vi "Read files V(Delay).vi"(10 "Path":path, 11 "Number":dbl) -> (3 "V":dbl format="%#_1g")   [LabVIEW 2020, in "GPP.lvlib"]
uses:
  GPP.lvlib
panel:
  out "V1":string
  out "Time":string
  out "LAST1":string
  out "Voltege":string
  out "ALL":string
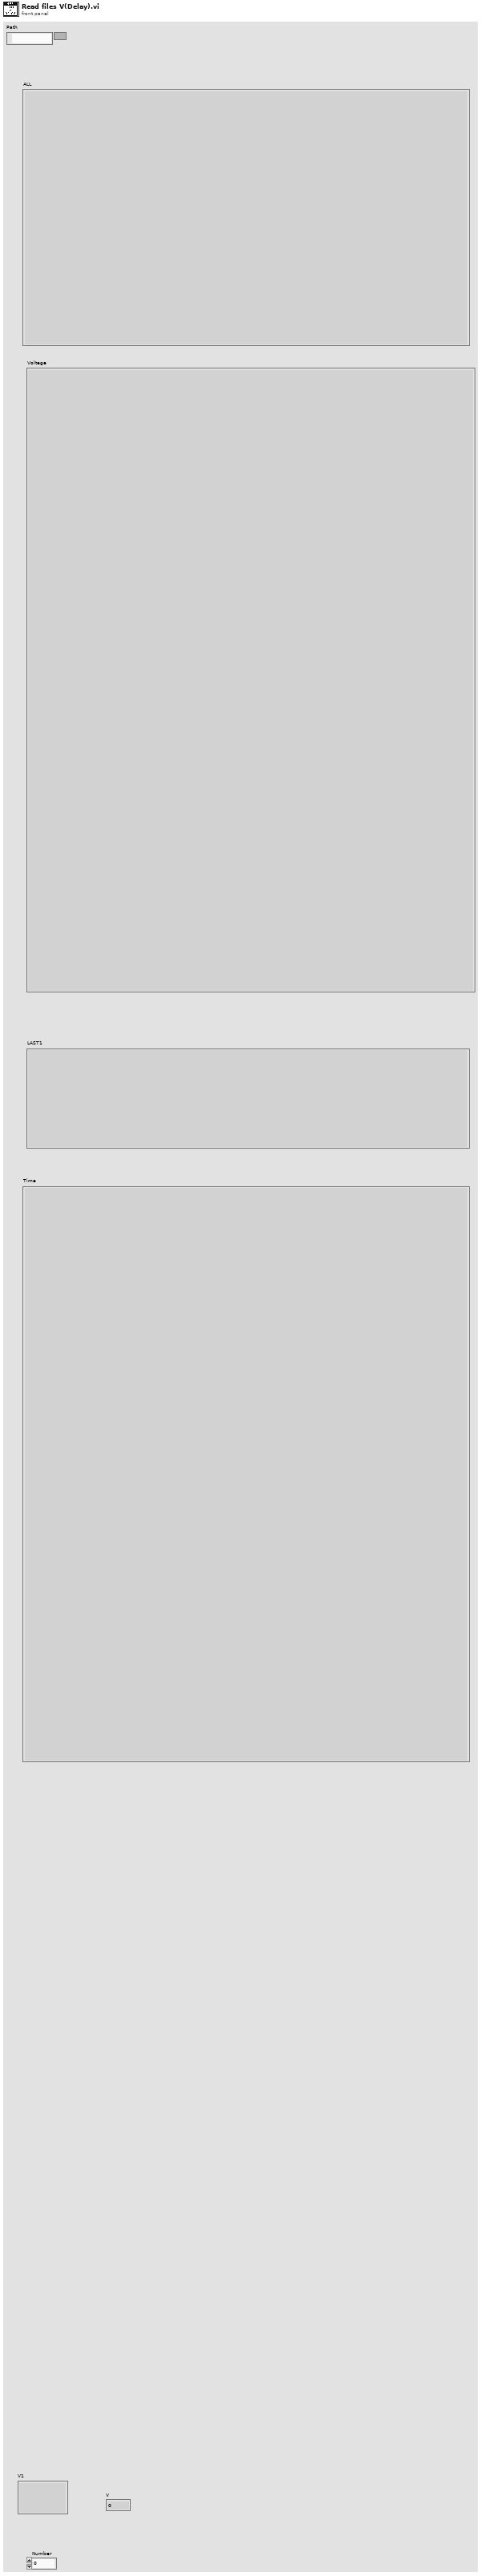
[diagram p1: front panel]
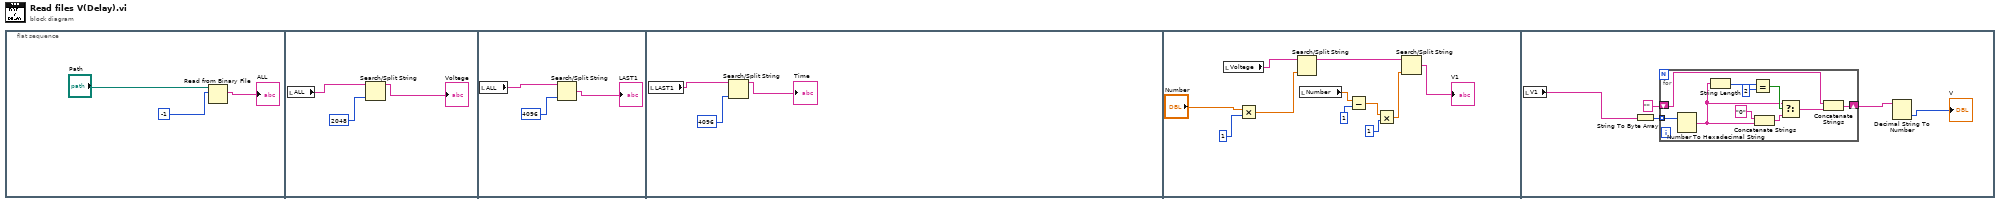
[diagram p0: block diagram]
diagram:
  n1 = flat-sequence {
    frame #0 {
      n2 = Read from Binary File(10:-1, 11:"Path") -> (2:→"ALL":string)  [unwired: 4 in, 3 out]
    }
    frame #1 {
      n3 = local read "ALL"() -> (w4:string)
      n4 = Search/Split String(string=w4, offset (0)=2048) -> (substring before match=→"Voltege":string)  [unwired: 1 in, 2 out]
    }
    frame #2 {
      n5 = local read "ALL"() -> (w7:string)
      n6 = Search/Split String(string=w7, offset (0)=4096) -> (match + rest of string=→"LAST1":string)  [unwired: 1 in, 2 out]
    }
    frame #3 {
      n7 = local read "LAST1"() -> (w10:string)
      n8 = Search/Split String(string=w10, offset (0)=4096) -> (substring before match=→"Time":string)  [unwired: 1 in, 2 out]
    }
    frame #4 {
      n9 = local read "Voltege"() -> (w13:string)
      n10 = Multiply(x="Number", y=1) -> (x*y=w16:dbl)
      n11 = Search/Split String(string=w13, offset (0)=w16) -> (substring before match=w17:string)  [unwired: 1 in, 2 out]
      n12 = local read "Number"() -> (w19:dbl)
      n13 = Subtract(x=w19, y=1) -> (x-y=w20:dbl)
      n14 = Multiply(x=w20, y=1) -> (x*y=w22:dbl)
      n15 = Search/Split String(string=w17, offset (0)=w22) -> (match + rest of string=→"V1":string)  [unwired: 1 in, 2 out]
    }
    frame #5 {
      n16 = local read "V1"() -> (w26:string)
      n17 = String To Byte Array(string=w26) -> (unsigned byte array=w27:u8[])
      n18 = for {
        tunnel: w27 -> [w38] mode=indexing
        shift-right: [w37] -> w25
        shift-left: "" -> [w36]
        n19 = Number To Hexadecimal String(2:w38) -> (0:w31:string)  [unwired: 1 in]
        n20 = String Length(string=w31) -> (length=w35:i32)
        n21 = Equal?(x=w35, y=2) -> (x = y?=w33:bool)
        n22 = Concatenate Strings("0" ("字符串"), w31) -> (w29:string)
        n23 = Select(t=w31, s=w33, f=w29) -> (s? t:f=w32:string)
        n24 = Concatenate Strings(w36, w32) -> (w37:string)
      }
      n25 = Decimal String To Number(string=w25) -> (number=→"V":i32)  [unwired: 2 in, 1 out]
    }
  }
